vi "Exponential.vi"   [LabVIEW 2017, in "NI_Matrix.lvlib"]
doc: "Computes the exponential of the input matrix."
uses:
  <vilib>/Analysis/Matrix/NI_Matrix.lvlib
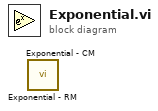
[diagram p0: block diagram]
diagram:
  n1 = call <vilib>:"Exponential - RM.vi"() -> ()  [unwired: 1 in, 1 out]
  n2 = call <vilib>:"Exponential - CM.vi"() -> ()  [unwired: 1 in, 1 out]
